vi "Example Loopback.vi"() -> ()   [LabVIEW 2010]
uses:
  C:/tf/play/labview/Tinkerforge.dll
  Tinkerforge.dll
panel:
  out "data":u8[](array[numeric])
  out "identifier":i64
  out "frameType":u8
  in  "stop":bool
  in  "uid":string="5556"
  in  "port":i32=4223
  in  "host":string="localhost"
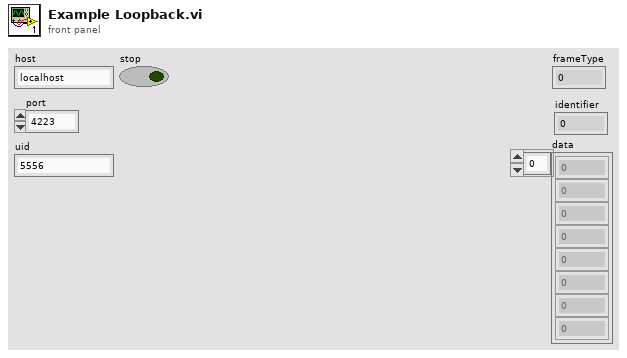
[diagram p1: front panel]
types:
  T1 = cluster{"data":u8[], "frameType":u8, "identifier":i64}
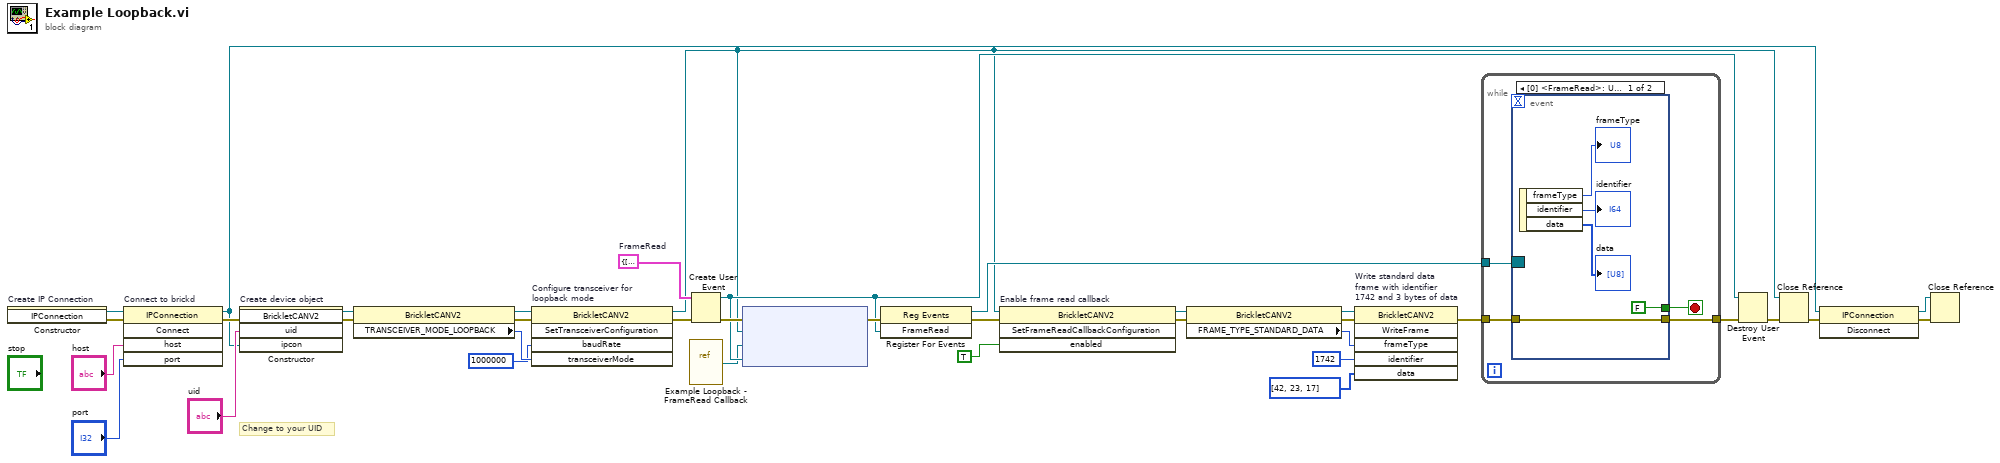
[diagram p0: block diagram]
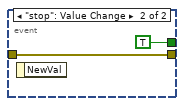
[diagram p2: hidden frame]
diagram:
  w20 = T1 {"data"=[], "frameType"=0, "identifier"=0}  # FrameRead
  # "Change to your UID"
  n1 = constructor on="Create IP Connection" class="IPConnection"() -> (reference out=w36:refnum<k24>, error out=w21:errorcluster)  [unwired: 3 in, 1 out]
  n2 = invoke on="Connect to brickd" class="IPConnection" method="Connect"(reference=w36, error in=w21, "host"="host", "port"="port") -> (reference out=w29:refnum<k24>, error out=w32:errorcluster)  [unwired: 1 in, 3 out]
  n3 = constructor on="Create device object" class="BrickletCANV2"(error in=w32, "uid"="uid", "ipcon"=w29) -> (reference out=w10:refnum<k24>, error out=w11:errorcluster)  [unwired: 2 in, 3 out]
  n4 = property class="BrickletCANV2"(reference=w10, error in=w11) -> (reference out=w5:refnum<k24>, error out=w6:errorcluster, "TRANSCEIVER_MODE_LOOPBACK"=w7:u8)
  n5 = invoke on="Configure transceiver for\nloopback mode" class="BrickletCANV2" method="SetTransceiverConfiguration"(reference=w5, error in=w6, "baudRate"=i64 1000000, "transceiverMode"=w7) -> (reference out=w9:refnum<k24>, error out=w8:errorcluster)  [unwired: 1 in, 3 out]
  n6 = vi-ref "Example Loopback - FrameRead Callback.vi"() -> ("vi reference"=w3:refnum<vi>)
  n7 = Create User Event(user event datatype=w20, error in=w8) -> (user event=w23:refnum<user-event>, error out=w27:errorcluster)
  n8 = node ("Register Event Callback")(w27, w9, w3, w23) -> (w26:errorcluster)  [unwired: 1 in, 1 out]
  n9 = register-events(error in=w26, w23) -> (reference out=w25:refnum<event-registration>, error out=w19:errorcluster)  [unwired: 1 in]
  n10 = invoke on="Enable frame read callback" class="BrickletCANV2" method="SetFrameReadCallbackConfiguration"(reference=w9, error in=w19, "enabled"=TRUE) -> (reference out=w17:refnum<k24>, error out=w15:errorcluster)  [unwired: 1 in, 2 out]
  n11 = property class="BrickletCANV2"(reference=w17, error in=w15) -> (reference out=w16:refnum<k24>, error out=w14:errorcluster, "FRAME_TYPE_STANDARD_DATA"=w13:u8)
  n12 = invoke on="Write standard data\nframe with identifier\n1742 and 3 bytes of data" class="BrickletCANV2" method="WriteFrame"(reference=w16, error in=w14, "frameType"=w13, "identifier"=i64 1742, "data"=u8[] [42, 23, 17]) -> (error out=w18:errorcluster)  [unwired: 1 in, 5 out]
  n13 = while {
    tunnel: w25 -> [w40]
    tunnel: [w39] -> w24
    tunnel: w18 -> [w38]
    stop <- w37 stop-if-true
    n14 = event shown="[0] <FrameRead>: User Event" {
      selector: w40 -> [_ _]
      dyn-events: _ -> [_ _]
      timeout: _ -> [_ _]
      tunnel: [w45 w46] -> w39
      tunnel: w38 -> [w45 w46]
      tunnel: [FALSE TRUE] -> w37
      event User Event {
        n15 = event-data() -> ("frameType"=→"frameType":u8, "identifier"=→"identifier":i64, "data"=→"data":u8[])  [unwired: 1 in]
      }
      event "stop": Value Change {
        n16 = event-data() -> ()  [unwired: 1 in, 1 out]
      }
    }
  }
  n17 = Destroy User Event(user event=w23, error in=w24) -> (error out=w22:errorcluster)
  n18 = Close Reference(reference=w9, error in (no error)=w22) -> (error out=w31:errorcluster)
  n19 = invoke class="IPConnection" method="Disconnect"(reference=w29, error in=w31) -> (reference out=w28:refnum<k24>, error out=w30:errorcluster)  [unwired: 1 in, 1 out]
  n20 = Close Reference(reference=w28, error in (no error)=w30) -> ()  [unwired: 1 out]
